vi "Dashboard Main.vi"() -> ()   [LabVIEW 2013]
uses:
  AnnieFramework/DoubleSolenoidAction.ctl
  AnnieFramework/CollectorAction.ctl
  AnnieFramework/CollectorWrapAction.ctl
  AnnieFramework/CatchAction.ctl
  AnnieFramework/AutoStates.ctl
  AnnieFramework/RollerAction.ctl
  AnnieFramework/AutoMode.ctl
  AnnieFramework/PassState.ctl
  AnnieFramework/HotGoalDetectType.ctl
  AnnieFramework/LowGoalState.ctl
  <vilib>/event_ctls.llb/eventvkey.ctl
  <vilib>/Rock Robotics/WPI/Dashboard/WPI_DashboardLogging Global.vi
  <vilib>/Utility/config.llb/Write Key (String).vi
  <vilib>/Utility/config.llb/Write Key (I32).vi
  KariFramework/CheckImageDistance.vi
  <vilib>/Utility/config.llb/NI_LVConfig.lvlib
panel:
  in  "Enable Vision":bool=TRUE
  out "Image Message":string="Timeout in Camera Communications"
  in  "Rec Mode":enum32{"Stop", "Record", "Playback"}(radio)
  in  "Dashboard Tab":T1(tab)
  out "Version":string
  in  "XBox":bool
  in  "DisableLCD":bool=TRUE
  out "GroundPassState":T2
  in  "DisableRollerOut":bool=TRUE
  out "FrontSonar":dbl
  out "ClosePressure":bool
  out "FarPressure":bool
  out "CatchState":T3
  out "CollectorWrapState":T4
  out "CollectorState":T5
  out "CollectorMotor":dbl
  out "ClapperState":T6
  out "RollerPneuState":T6
  out "FiringCylinder2":bool
  out "FiringCylinder1":bool
  out "Kicker":bool
  out "AutoDistanceDone?":bool
  out "BackSonar":dbl
  out "BottomLS":bool
  out "TopLS":bool
  in  "MaxMotorChange":dbl=1.5
  out "Error":bool
  out "Right Motor":dbl
  out "Left Motor":dbl
  in  "Camera Settings":T7={"Frame Rate"=30, "Compression"=30, "Size"=1} {"Frame Rate" scale=1.0..30.0; "Size" items=["640x480", "320x240", "160x120"]}
  out "Mode":T8(ring)=enum."Auto Disabled"
  out "Camera IP":string
  in  "DB Camera Config":bool
  out "fps":dbl format="%#.1g"
  out "Mbps":dbl format="%#.1g"
  out "Mbps 2":bool
  out "CloseDist":bool
  out "FarDist":bool
  out "Pressure":dbl
  out "RollerMotorState":T9
  in  "DisableServo":bool=TRUE
  out "ElevatedPassState":T2
  out "Arcade":bool
  out "TankDriveTime":dbl
  out "SonicShifter":bool
  out "StraightDrive":bool
  out "HalfDrive":bool
  out "ReverseDrive":bool
  out "Enum":T10
  in  "BallSettleWait":i32=130
  in  "PreCheckGoalWait":i32=260
  in  "Slowdown":dbl=36.0
  in  "Brake":dbl=12.0
  in  "DriveDistance":dbl=36.0
  in  "DriveMinTime":i32=2000
  in  "DriveTimeout":i32=5000
  out "WasHot?":bool
  out "DriveTimeOut":bool
  out "CheckGoalTimedOut?":bool
  out "ElapsedTime":u32
  out "StateTime":u32
  out "CurrentState":T11
  out "RaiseArmTimedOut":bool
  out "LowerArmTimedOut":bool
  out "IDMatched?":bool
  in  "AutoID":i32=3061
  in  "AutoMode":T12=enum."OneBallCollector"
  in  "WebcamStartTime (ms)":i32=2000
  out "WebcamMatched?":bool
  in  "SaveToDisk?":bool
  in  "WebcamImages":i32=1
  in  "ResetWebcam?":bool=TRUE
  out "WebcamImagesProcessed":i32
  in  "HotGoalType":T13
  out "ServoAngle":dbl
  in  "% Cutoff":dbl=0.5
  out "NumHot":i32
  out "NumProcessed":i32
  in  "NumSamples":i32=5
  out "ProcessImage?":bool
  in  "Finished?":bool
  in  "Hot?":bool
  in  "Score cutoff":dbl=0.5
  in  "Color System":u16(ring)=2 items=["RGB", "HSL", "HSV", "HSI"]
  out "Distance (ft)":dbl
  in  "Color Components":T14={"Hue"={112.0, 144.0}, "Sat"={202.0, 255.0}, "Val"={237.0, 255.0}} {"Val" scale=0.0..255.0; "Sat" scale=0.0..255.0; "Hue" scale=0.0..255.0 scale format="%#_3g"}
  out "LoopTime":u32
  in  "Calibrate?":bool
  in  "Reset?":bool
  in  "Test Slider":dbl(slide) scale=0.0..100.0 scale format="%#_3g"
  in  "On/Off":bool caption="Solenoid"
  in  "Test Name":u16(ring) items=["Select the test to run...", "Example Test", "-------------------------------", "List of tests is built in robot code.", "Replace with your own automated tests."]
  in  "Test Tree":string(tree)
  in  "Motor":cluster{"Value":dbl, "Enable":bool} {"Value" scale=-1.0..1.0 scale format="%#_3g"}
  out "Progress":T15 {"Test Progress" scale=0.0..100.0}
  in  "Rev/Fwd":cluster{"Forward":bool, "Reverse":bool}
  in  "Test Ring":u16(ring) items=["Auto", "Fixed indoor", "Fixed outdoor 1", "Fixed outdoor 2", "Fixed fluorescent 1", "Fixed fluorescent 2", "Hold current"]
  in  "Listbox":i32(listbox)
  out "Tree":string(tree)
  out "Timer":u32
  in  "CountdownStartTime":u32=10
  in  "AutoLength":u32=10
  in  "TeleopLength":u32=140
  out "Status":T16(ring)
  out "Errors":T17(array[cluster])
  in  "Reset":bool
  out "Camera Image":T18(plugin-control)
  # "DRIVE"
  # "GENERAL"
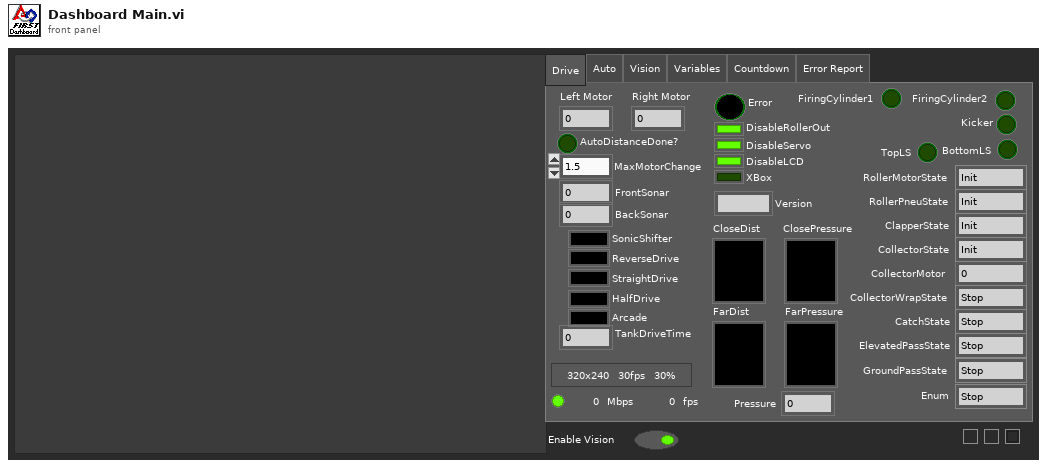
[diagram p1: front panel]
types:
  T1 = enum32{"Drive", "Auto", "Vision", "Test", "Checklist", "Variables", "Countdown", "Error Report"}
  T2 = typedef "PassState.ctl" = enum16{"Stop", "Pass"}
  T3 = typedef "CatchAction.ctl" = enum16{"Stop", "PreCatch", "Catch"}
  T4 = typedef "CollectorWrapAction.ctl" = enum16{"Stop", "PreCollect", "Collect"}
  T5 = typedef "CollectorAction.ctl" = enum16{"Init", "Raise", "Lower", "Stop", "GetStatus"}
  T6 = typedef "DoubleSolenoidAction.ctl" = enum16{"Init", "Middle", "In", "Out"}
  T7 = cluster{"Frame Rate":i32, "Compression":i32, "Size":u16}
  T8 = enum8{"Tele-Op Disabled", "Tele-Op Enabled", "Auto Disabled", "Auto Enabled", "Test Disabled", "Test Enabled", ""}
  T9 = typedef "RollerAction.ctl" = enum16{"Init", "Off", "Forward", "Reverse"}
  T10 = typedef "LowGoalState.ctl" = enum16{"Stop", "Shoot"}
  T11 = typedef "AutoStates.ctl" = enum16{"Init", "LowerArmCheckGoal", "DriveBack", "Collect", "StopCollect", "LiftArm", "RaiseServo", "Drive", "ShootCollectorUp", "RaiseArm", "ShootCollectorDown", "Rotate1", "Rotate2", "Stop"}
  T12 = typedef "AutoMode.ctl" = enum16{"OneBallFront", "OneBallCollector", "TwoBallNormal", "TwoBallHot"}
  T13 = typedef "HotGoalDetectType.ctl" = enum16{"VisionTarget", "Kinect"}
  T14 = cluster{"Hue":cluster{dbl, dbl}, "Sat":cluster{dbl, dbl}, "Val":cluster{dbl, dbl}}
  T15 = cluster{"Test Progress":u8, "Test Progress Text":string}
  T16 = enum8{"Disconnected", "E-Stop", "Disabled", "Enabled"}
  T17 = cluster{"status":bool, "code":i32, "location":string, "source":string}[]
  T18 = typedef "IMAQ Image.ctl" = refnum<image>
  T19 = enum32{"Drive", "Operation", "Auto", "Test", "Checklist", "Variables"}
  T20 = typedef "Image Type" = u32
  T21 = typedef "NI_LVConfig.lvlib/Config Data RefNum.ctl" = refnum<k1>
  T22 = cluster{"Digital Inputs":bool[], "Digital Outputs":bool[]}
  T23 = cluster{"Competition mode":bool, "Robot Link":bool, "Autonomous":bool, "Enabled":bool, "E-Stop":bool, "Simulated":bool, "TestMode":bool, "Docked Window":bool}
  T24 = typedef "CountdownAction.ctl" = enum16{"Start", "Reset", "Continue", "Idle"}
  T25 = cluster{"Boolean":bool, "Numeric":i32, "String":string, "String":string}[]
  T26 = cluster{cluster{dbl, dbl}, cluster{dbl, dbl}, cluster{dbl, dbl}}
  T27 = typedef "Sound Output Task ID.ctl" = u32
  T28 = typedef "eventvkey.ctl" = enum16{"ASCII", "Enter", "Return", "Shift", "Ctrl", "Alt", "Cmd", "Opt", "Caps", "NumLock", "Clear", "Break", "Up", "Down", "Left", "Right", "Insert", "Delete", "Home", "End", "PageUp", "PageDown", "Escape", "Help", "Pause", "ScrollLock", "F1", "F2", "F3", "F4", "F5", "F6", "F7", "F8", "F9", "F10", "F11", "F12", "F13", "F14", "F15", "F16", "F17", "F18", "F19", "F20", "F21", "F22", "F23", "F24", "Play", "VolumeUp", "VolumeDown", "Mute", "Two Byte Char"}
  T29 = cluster{"Image Size":bool, "Image Type":bool, "Pixel Value":bool, "ROI Information":bool, "Zoom Factor":bool}
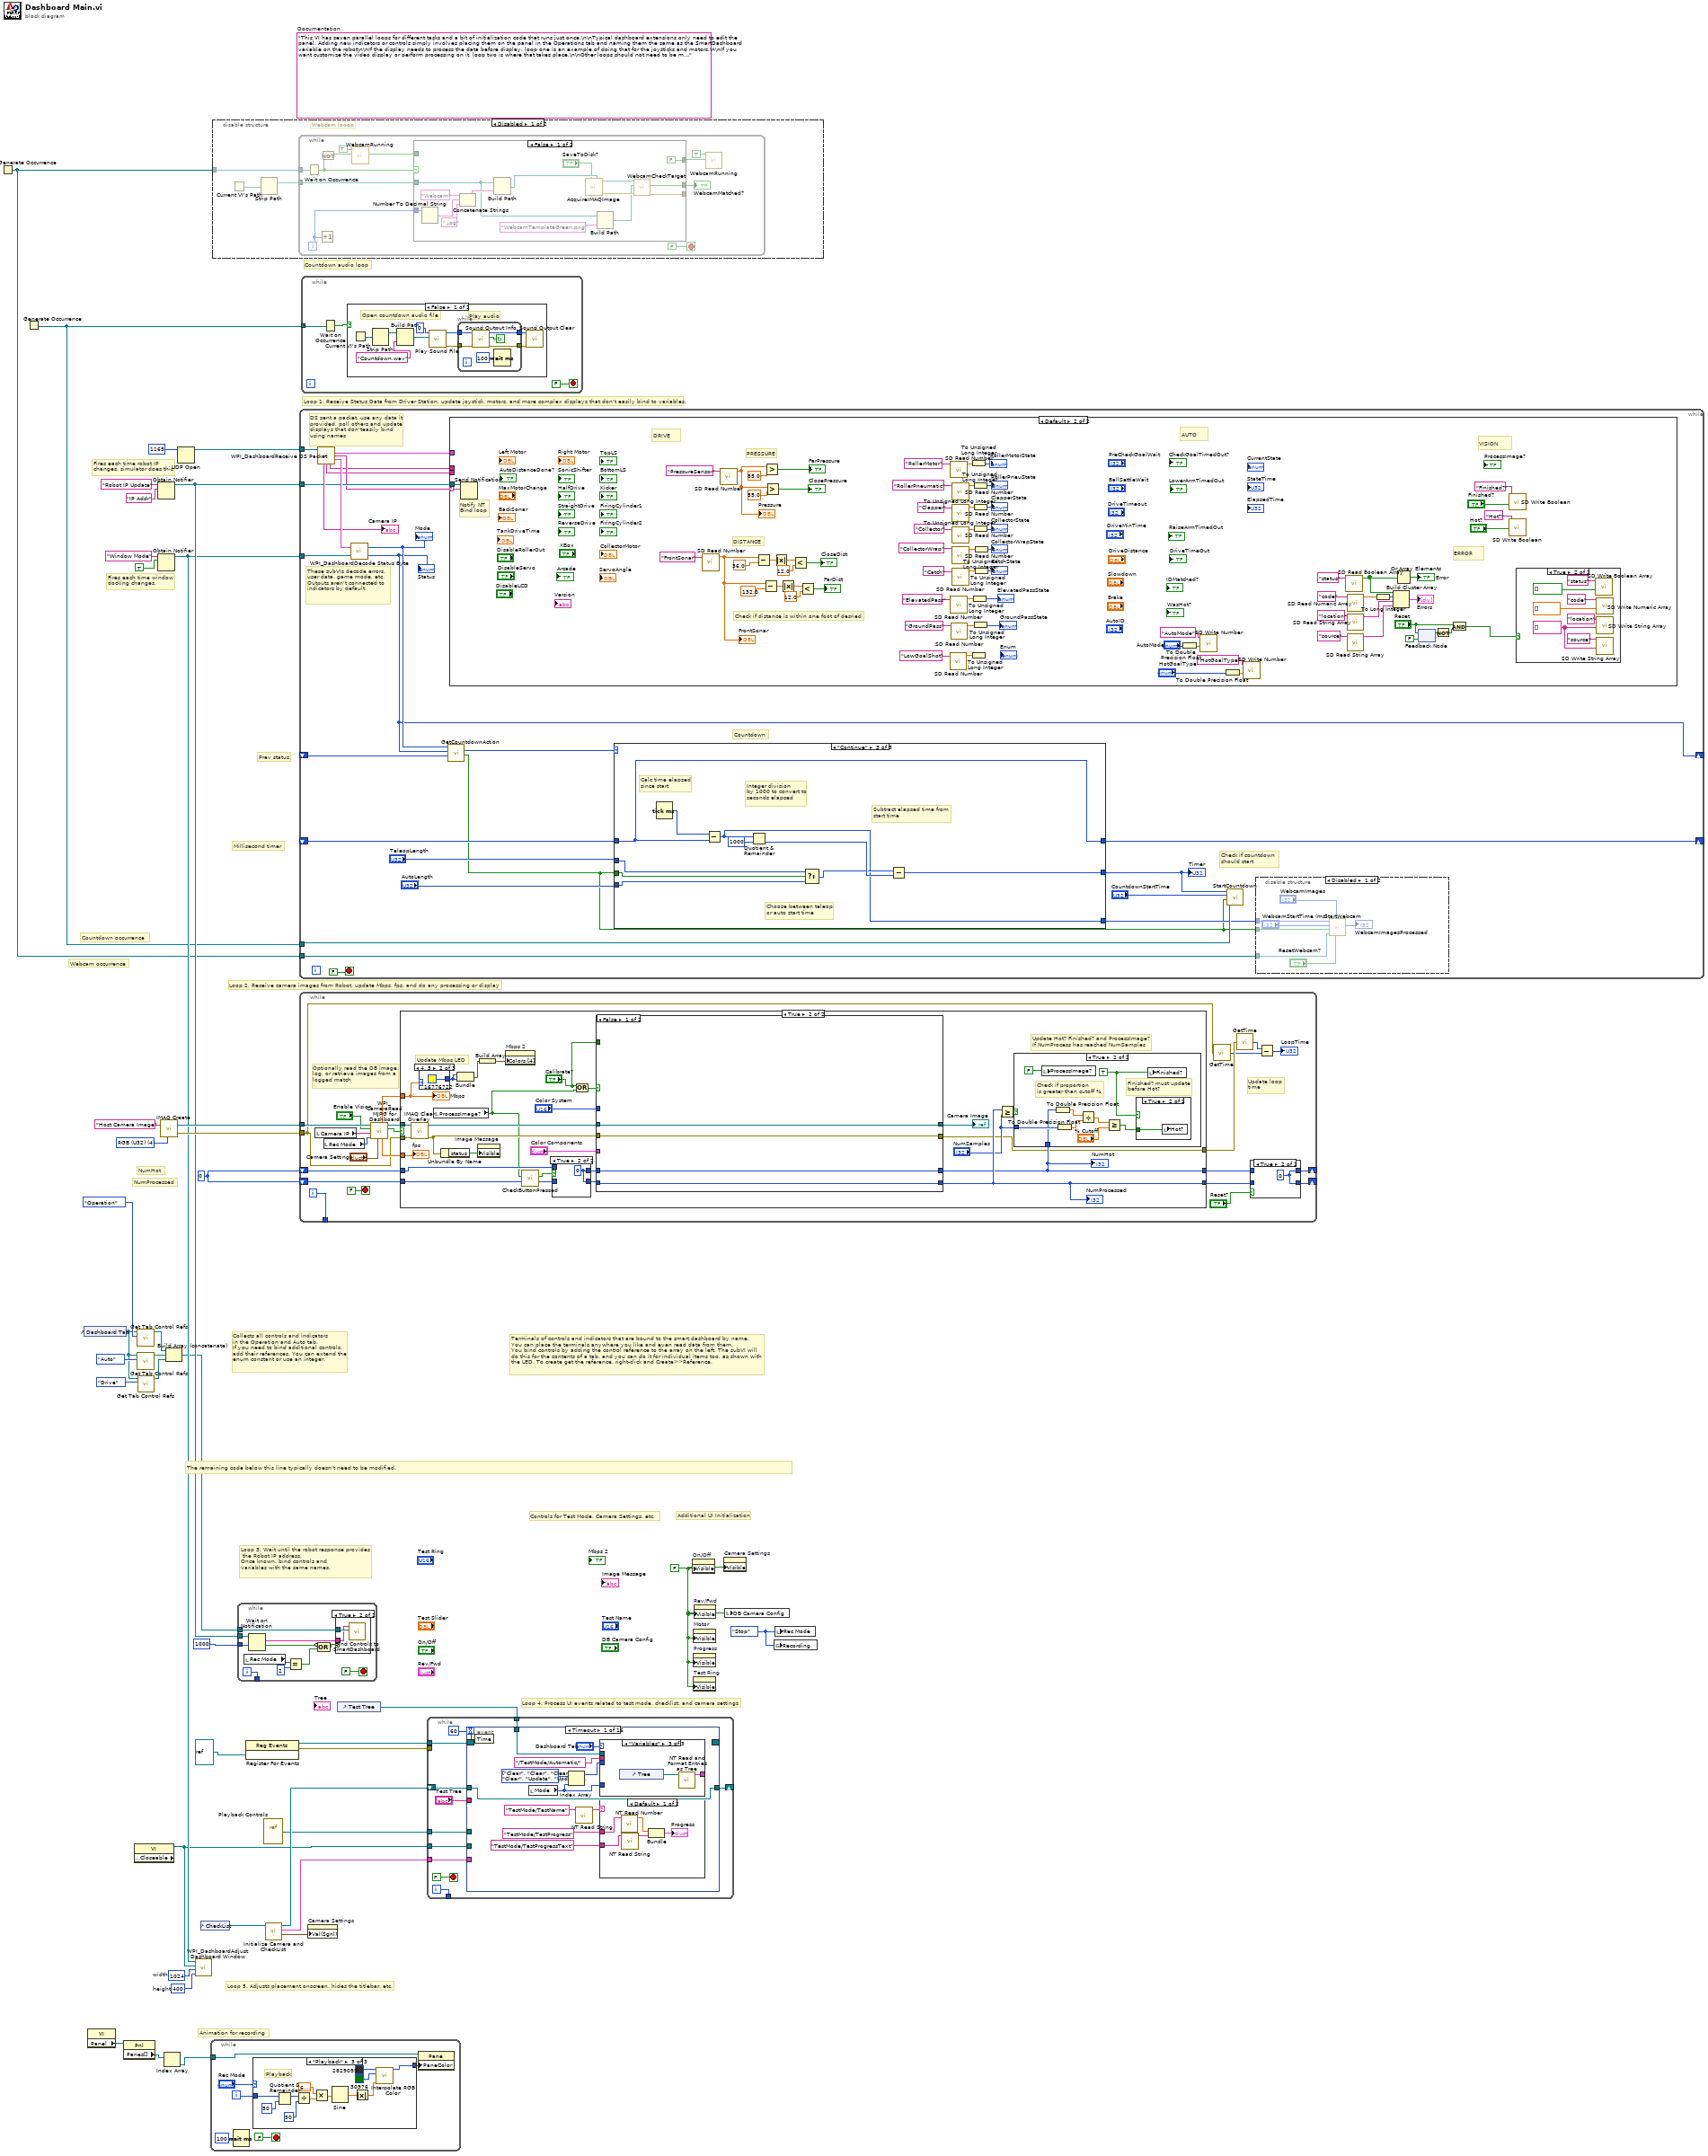
[diagram p0: block diagram]
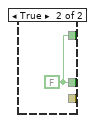
[diagram p2: hidden frame]
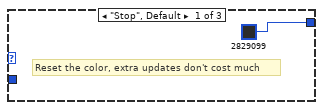
[diagram p5: hidden frame]
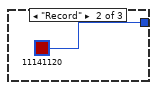
[diagram p6: hidden frame]
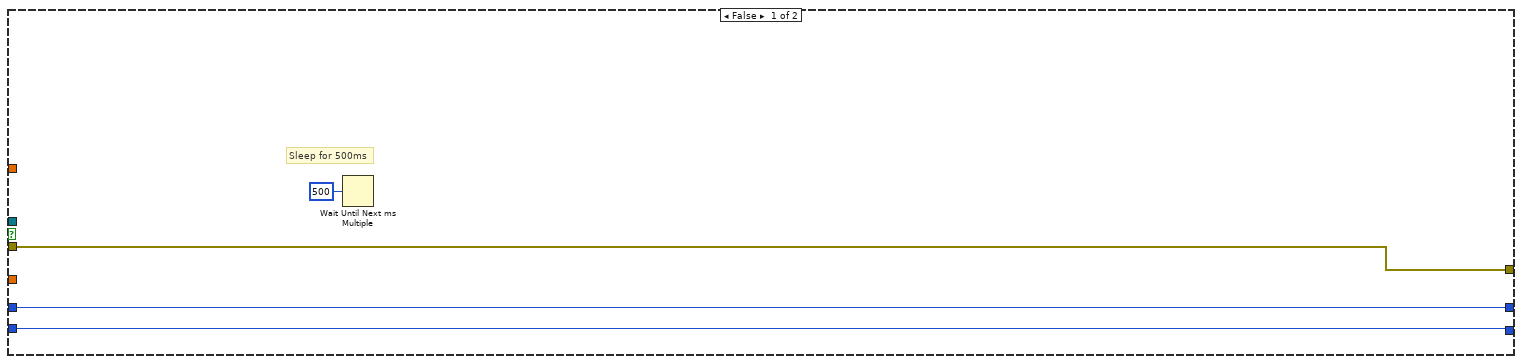
[diagram p9: hidden frame]
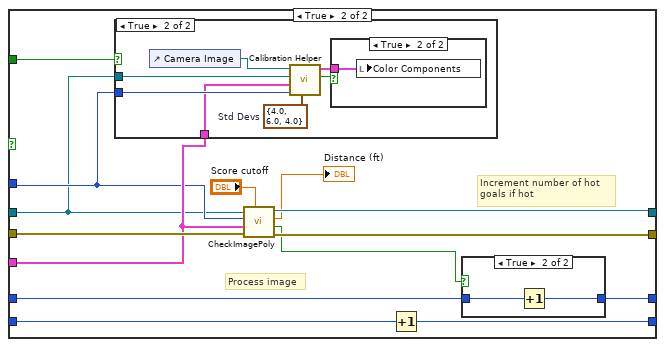
[diagram p13: hidden frame]
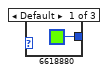
[diagram p17: hidden frame]
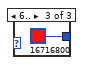
[diagram p18: hidden frame]
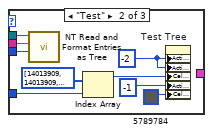
[diagram p20: hidden frame]
diagram:
  w3 = 0
  w12 = enum32{"Stop", "Record", "Playback"}."Stop" ("Rec Mode")
  w15 = 400  # height
  w16 = 1024  # width
  w29 = FALSE ("Visible")
  (unwired) "This VI has seven parallel loops for different tasks and a bit of initialization code that runs just once.\n\nTypical dashboard extensions only need to edit the panel. Adding new indicators or controls simply involves placing them on the panel in the Operations tab and naming them the same as the SmartDashboard variable on the robot\n\nIf the display needs to process the data before display, loop one is an example of doing that for the joysticks and motors.\n\nIf you want customize the video display or perform processing on it, loop two is where that takes place.\n\nOther loops should not need to be modified. They are pretty standard, and document the task they perform."  # Documentation
  w39 = T20 4 items=["Grayscale (U8)", "Grayscale (I16)", "Grayscale (SGL)", "Complex (CSG)", "RGB (U32)", "HSL (U32)", "RGB (U64)"] ("Image Type")
  # "Webcam occurrence"
  # "Countdown audio loop"
  # "Countdown occurrence"
  # "Millisecond timer"
  # "Prev status"
  # "NumProcessed"
  # "NumHot"
  # "Controls for Test Mode, Camera Settings, etc."
  # "Additional UI Initialization"
  # "Animation for recording"
  # "Fires each time robot IP\nchanges, simulator does this"
  # "Fires each time window\ndocking changes."
  # "Collects all controls and indicators\nin the Operation and Auto tab.\nIf you need to bind additional controls,\nadd their references. You can extend the\nenum constant or use an integer."
  # "The remaining code below this line typically doesn't need to be modified."
  # "Loop 4. Process UI events related to test mode, checklist, and camera settings"
  # "Terminals of controls and indicators that are bound to the smart dashboard by name.\nYou can place the terminals anywhere you like and even read data from them.\nYou bind controls by adding the control reference to the array on the left. The subVI will\ndo this for the contents of a tab, and you can do it for individual items too, as shown with\nthe LED. To create get the reference, right-click and Create>>Reference."
  # "Loop 3. Wait until the robot response provides\n the Robot IP address.\nOnce known, bind controls and\nvariables with the same names."
  # "Loop 5. Adjusts placement onscreen, hides the titlebar, etc."
  # "Loop 1. Receive Status Data from Driver Station, update joystick, motors, and more complex displays that don't easily bind to variables."
  # "Loop 2. Receive camera images from Robot, update Mbps, fps, and do any processing or display"
  n1 = Generate Occurrence() -> (w1:refnum<k4>)
  n2 = Generate Occurrence() -> (w2:refnum<k4>)
  n3 = control-ref of="Dashboard Tab"() -> (w5:refnum<vi>)
  n4 = property class="VI"() -> ("Panel"=w23:refnum<vi>)  [unwired: 2 in, 2 out]
  n5 = property class="Pnl"(reference=w23) -> ("Panes[]"=w24:refnum<vi>[])  [unwired: 1 in, 2 out]
  n6 = property class="VI" props=["Front Panel.Closeable"]() -> (reference out=w11:refnum<vi>)  [unwired: 2 in, 2 out]
  n7 = call <vilib>:"Get Tab Control Refs.vi"("Page Index"=T19."Operation" ("Dashboard Tab"), "TabControl in"=w5) -> ("ControlsOnPage"=w9:refnum<vi>[])  [unwired: 9 in]
  n8 = call <vilib>:"Get Tab Control Refs.vi"("Page Index"=T19."Auto" ("Dashboard Tab"), "TabControl in"=w5) -> ("ControlsOnPage"=w10:refnum<vi>[])  [unwired: 9 in]
  n9 = call <vilib>:"Get Tab Control Refs.vi"("Page Index"=T19."Drive" ("Dashboard Tab"), "TabControl in"=w5) -> ("ControlsOnPage"=w4:refnum<vi>[])  [unwired: 9 in]
  n10 = Obtain Notifier(name (unnamed)="Robot IP Update", notification data type="IP Addr" ("name (unnamed)")) -> (notifier out=w33:refnum<notifier>)  [unwired: 2 in, 2 out]
  n11 = Obtain Notifier(name (unnamed)="Window Mode", notification data type=TRUE) -> (notifier out=w14:refnum<notifier>)  [unwired: 2 in, 2 out]
  n12 = call "IMAQ Create"("Image Name"="Host Camera Image", "Image Type"=w39) -> ("New Image"=w37:T18, "error out"=w36:errorcluster)  [unwired: 2 in, 1 out]
  n13 = Index Array(array=w24) -> (element=w22:refnum<vi>)  [unwired: 1 in]
  n14 = Build Array (concatenate)(w9, w10, w4) -> (w8:refnum<vi>[])
  n15 = UDP Open(11:u16 1165 ("port")) -> (port=w40:refnum<k16>)  [unwired: 2 in, 4 out]
  n16 = call <vilib>:"WPI_DashboardAdjust Dashboard Window.vi"("height"=w15, "width"=w16, "reference in"=w11, "Notifier in"=w14) -> ()  [unwired: 8 in]
  n17 = control-ref of="CheckList"() -> (w13:refnum<vi>)
  n18 = while {
    tunnel: w22 -> [w43]
    i -> [w46]
    stop <- FALSE stop-if-true
    n19 = Wait (ms)(milliseconds to wait=u32 100) -> ()  [unwired: 1 out]
    n20 = case shown="\"Playback\"" "Rec Mode" {
      tunnel: w46 -> [_ _ w61]
      tunnel: [u32 2829099 ("Base Color") u32 11141120 ("Target Color") w50] -> w42
      frame "Stop", Default {
        # "Reset the color, extra updates don't cost much"
      }
      frame "Record" {
      }
      frame "Playback" {
        # "Playback"
        n21 = Quotient & Remainder(x=w61, y=u32 50 ("milliseconds to wait")) -> (x-y*floor(x/y)=w57:u32)  [unwired: 1 out]
        n22 = Divide(x=w57, y=u32 50 ("milliseconds to wait")) -> (x/y=w54:dbl)
        n23 = Multiply(x=6.283185307179586, y=w54) -> (x*y=w59:dbl)
        n24 = Sine(x=w59) -> (sin(x)=w58:dbl)
        n25 = Absolute Value(x=w58) -> (abs(x)=w51:dbl)
        n26 = call "Interpolate RGB Color.vi"("Proportion"=w51, "Target Color"=u32 30976, "Base Color"=u32 2829099) -> ("Result Color"=w50:u32)  [unwired: 8 in]
      }
    }
    n27 = property class="Pane"(reference=w43, "PaneColor"=w42) -> ()  [unwired: 1 in, 2 out]
  }
  n28 = disable-structure shown="Disabled" {
    disable-tunnel: w1 -> [w64 _]
    frame Disabled {
      # "Webcam looop"
      n29 = Current VI's Path() -> (path=w63:path)
      n30 = Strip Path(path=w63) -> (stripped path=w62:path)  [unwired: 1 out]
      n31 = while {
        tunnel: w64 -> [w75]
        tunnel: w62 -> [w72]
        i -> [w71]
        stop <- FALSE stop-if-true
        n32 = Wait on Occurrence(2:w75) -> (0:w69:bool)  [unwired: 2 in]
        n33 = Increment(x=w71) -> ()  [unwired: 1 out]
        n34 = Not(x=w69) -> (.not. x?=w68:bool)
        n35 = call "WebcamRunning"("NewValue"=w68, "Write?"=TRUE) -> ("CurrentValue"=w65:bool)  [unwired: 9 in]
        n36 = case shown="False" w69 {
          tunnel: [w88 _] -> _
          tunnel: [w87 w91] -> w73
          tunnel: w71 -> [w85 _]
          tunnel: w72 -> [w79 _]
          tunnel: [FALSE w91] -> w66
          tunnel: w65 -> [_ _]
          frame False {
            n37 = Number To Decimal String(number=w85) -> (decimal integer string=w84:string)  [unwired: 1 in]
            n38 = Concatenate Strings("Webcam", w84, ".jpg" ("string")) -> (w83:string)
            n39 = Build Path(base path=w79, name or relative path=w83) -> (appended path=w82:path)
            n40 = call "AcquireIMAQImage.vi"("ImagePath"=w82, "SaveToDisk?"="SaveToDisk?") -> ("error out"=w89:errorcluster, "ImageOut"=w90:T18)  [unwired: 8 in]
            n41 = Build Path(base path=w79, name or relative path="WebcamTemplateGreen.png") -> (appended path=w78:path)
            n42 = call "WebcamCheckTarget.vi"("error in"=w89, "TemplatePath"=w78, "ImageIn"=w90) -> ("error out"=w88:errorcluster, "MatchFound?"=w87:bool)  [unwired: 6 in, 1 out]
          }
          frame True {
            w91 = FALSE ("MatchFound?")
          }
        }
        "WebcamMatched?" <- w73
        n43 = call "WebcamRunning"("NewValue"=w66, "Write?"=TRUE) -> ()  [unwired: 9 in, 1 out]
      }
    }
    frame Enabled {
    }
  }
  n44 = while {
    tunnel: w8 -> [w102]
    tunnel: w33 -> [w100]
    tunnel: [w98] -> _
    tunnel: u32 1000 ("milliseconds to wait") -> [w97]
    i -> [w98]
    stop <- FALSE stop-if-true
    n45 = local read "Rec Mode"() -> (w93:enum32{"Stop", "Record", "Playback"})
    n46 = Wait on Notification(notifier=w100, timeout in ms (-1)=w97) -> (notification=w99:string, timed out?=w95:bool)  [unwired: 2 in, 2 out]
    n47 = Equal?(x=w93, y=u16 2 ("Rec Mode")) -> (x = y?=w94:bool)
    n48 = Compound Arithmetic op=OR(invert w95, w94) -> (w96:bool)
    n49 = case shown="True" w96 {
      tunnel: w102 -> [_ w104]
      tunnel: w99 -> [_ w103]
      frame False {
      }
      frame True {
        n50 = call <vilib>:"Bind Controls to SmartDashboard.vi"("Bound Control Refs"=w104, "Server IP Address"=w103) -> ()  [unwired: 10 in]
      }
    }
  }
  n51 = register-events(refnum<vi> refnum) -> (reference out=w20:refnum<event-registration>, error out=w19:errorcluster)  [unwired: 2 in]
  n52 = vi-ref "Playback Controls.vi"() -> (w21:refnum<vi>)
  n53 = call "Initialize Camera and CheckList.vi"("ListBox in"=w13) -> ("Cluster"=w27:cluster{"value":i32, "value":i32, "index":i32}, "Array"=w28:cluster{string[]}[], "File Refnum"=w26:T21)  [unwired: 8 in]
  n54 = while {
    tunnel: w40 -> [w126]
    tunnel: w33 -> [w123]
    tunnel: w14 -> [w125]
    shift-right: [w117] -> _
    shift-left: _ -> [w116]
    shift-right: [w114] -> _
    shift-left: _ -> [w113]
    tunnel: w2 -> [w108]
    tunnel: w1 -> [w105]
    stop <- FALSE stop-if-true
    # "Check if countdown\nshould start"
    # "Countdown"
    # "DS sent a packet. use any data it\nprovided, poll others and update\ndisplays that don'teasily bind\nusing names"
    # "These subVIs decode errors, user data, game mode, etc.\nOutputs aren't connected to indicators by default"
    n55 = call <vilib>:"WPI_DashboardReceive DS Packet.vi"("Recv Socket"=w126) -> ("Driver Station"=w119:T22, "Robot IP Address"=w122:string, "Status"=w127:T23, "Camera IP Address"=→"Camera IP":string, "Low Priority User Data"=w121:string, "High Priority User Data"=w120:string)  [unwired: 1 in, 8 out]
    n56 = call <vilib>:"WPI_DashboardDecode Status Byte.vi"("Window Mode Notifier"=w125, "Status"=w127) -> ("Status"=w117:T16, "Mode"=w118:T8)
    "Mode" <- w118
    "Status" <- w117
    n57 = call "GetCountdownAction.vi"("PrevStatus"=w116, "CurrentStatus"=w117, "CurrentMode"=w118) -> ("Teleop?"=w106:bool, "Action"=w115:T24)  [unwired: 7 in]
    n58 = case shown="Default" w122 {
      selector: w122 -> [_ w224]
      tunnel: w123 -> [_ w225]
      tunnel: w121 -> [_ _]
      tunnel: w120 -> [_ _]
      tunnel: w119 -> [_ _]
      frame "0.0.0.0" {
        # "DS not sending packets, or no robot exists yet.\nDon't poll the variables"
      }
      frame Default {
        # "Check if distance is within one foot of desried"
        # "ERROR"
        # "DISTANCE"
        # "PRESSURE"
        # "VISION"
        # "AUTO"
        # "DRIVE"
        # "Notify NT\nBind loop"
        n59 = Send Notification(notification=w224, notifier=w225) -> ()  [unwired: 1 in, 2 out]
        n60 = call <vilib>:"SD Read Number.vi"("Name"="FrontSonar") -> ("Numeric"=w172:dbl)  [unwired: 8 in, 2 out]
        "FrontSonar" <- w172
        n61 = call <vilib>:"SD Read Number.vi"("Name"="PressureSensor") -> ("Numeric"=w171:dbl)  [unwired: 8 in, 2 out]
        "Pressure" <- w171
        n62 = Subtract(x=w172, y=36.0) -> (x-y=w181:dbl)
        n63 = Subtract(x=w172, y=132.0) -> (x-y=w175:dbl)
        n64 = Greater?(x=w171, y=85.0) -> (0:→"FarPressure":bool)
        n65 = Greater?(x=w171, y=55.0) -> (0:→"ClosePressure":bool)
        n66 = Absolute Value(x=w181) -> (abs(x)=w180:dbl)
        n67 = Absolute Value(x=w175) -> (abs(x)=w176:dbl)
        n68 = Less?(x=w180, y=12.0) -> (x < y?=→"CloseDist":bool)
        n69 = Less?(x=w176, y=12.0) -> (x < y?=→"FarDist":bool)
        n70 = call <vilib>:"SD Read Number.vi"("Name"="LowGoalShot") -> ("Numeric"=w154:dbl)  [unwired: 8 in, 2 out]
        n71 = call <vilib>:"SD Read Number.vi"("Name"="RollerMotor") -> ("Numeric"=w169:dbl)  [unwired: 8 in, 2 out]
        n72 = call <vilib>:"SD Read Number.vi"("Name"="ElevatedPass") -> ("Numeric"=w163:dbl)  [unwired: 8 in, 2 out]
        n73 = call <vilib>:"SD Read Number.vi"("Name"="GroundPass") -> ("Numeric"=w162:dbl)  [unwired: 8 in, 2 out]
        n74 = call <vilib>:"SD Read Number.vi"("Name"="RollerPneumatic") -> ("Numeric"=w202:dbl)  [unwired: 8 in, 2 out]
        n75 = call <vilib>:"SD Read Number.vi"("Name"="Clapper") -> ("Numeric"=w200:dbl)  [unwired: 8 in, 2 out]
        n76 = call <vilib>:"SD Read Number.vi"("Name"="Collector") -> ("Numeric"=w197:dbl)  [unwired: 8 in, 2 out]
        n77 = call <vilib>:"SD Read Number.vi"("Name"="CollectorWrap") -> ("Numeric"=w194:dbl)  [unwired: 8 in, 2 out]
        n78 = call <vilib>:"SD Read Number.vi"("Name"="Catch") -> ("Numeric"=w191:dbl)  [unwired: 8 in, 2 out]
        n79 = To Unsigned Long Integer(number=w169) -> (unsigned 32bit integer=→"RollerMotorState":u32)
        n80 = To Unsigned Long Integer(number=w154) -> ()  [unwired: 1 out]
        n81 = To Unsigned Long Integer(number=w163) -> (unsigned 32bit integer=→"ElevatedPassState":u32)
        n82 = To Unsigned Long Integer(number=w202) -> (unsigned 32bit integer=→"RollerPneuState":u32)
        n83 = To Unsigned Long Integer(number=w200) -> (unsigned 32bit integer=→"ClapperState":u32)
        n84 = To Unsigned Long Integer(number=w162) -> (unsigned 32bit integer=→"GroundPassState":u32)
        n85 = To Unsigned Long Integer(number=w197) -> (unsigned 32bit integer=→"CollectorState":u32)
        n86 = To Unsigned Long Integer(number=w194) -> (unsigned 32bit integer=→"CollectorWrapState":u32)
        n87 = To Unsigned Long Integer(number=w191) -> (unsigned 32bit integer=→"CatchState":u32)
        n88 = To Double Precision Float(number="AutoMode") -> (double precision float=w165:dbl)
        n89 = call <vilib>:"SD Write Number.vi"("Numeric"=w165, "Name"="AutoMode") -> ()  [unwired: 8 in, 2 out]
        n90 = To Double Precision Float(number="HotGoalType") -> (double precision float=w158:dbl)
        n91 = call <vilib>:"SD Write Number.vi"("Numeric"=w158, "Name"="HotGoalType") -> ()  [unwired: 8 in, 2 out]
        n92 = call <vilib>:"SD Read Boolean Array.vi"("Name"="status") -> ("Boolean Array"=w213:bool[])  [unwired: 8 in, 2 out]
        n93 = call <vilib>:"SD Read Numeric Array.vi"("Name"="code") -> ("Numeric Array"=w212:dbl[])  [unwired: 8 in, 2 out]
        n94 = call <vilib>:"SD Read String Array.vi"("Name"="location") -> ("String Array"=w211:string[])  [unwired: 9 in, 1 out]
        n95 = call <vilib>:"SD Read String Array.vi"("Name"="source") -> ("String Array"=w210:string[])  [unwired: 9 in, 1 out]
        n96 = To Long Integer(number=w212) -> (32bit integer=w218:i32[])
        n97 = Build Cluster Array(w213, w218, w211, w210) -> (→"Errors":T25)
        n98 = Or Array Elements(Boolean array=w213) -> (logical OR=→"Error":bool)
        n99 = feedback #1(FALSE ("Reset")) -> (w221:bool)
        n100 = feedback-in #1("Reset") -> ()
        n101 = Not(x=w221) -> (.not. x?=w220:bool)
        n102 = And(x="Reset", y=w220) -> (x .and. y?=w219:bool)
        n103 = call <vilib>:"SD Write Boolean.vi"("Boolean"="Finished?", "Name"="Finished?") -> ()  [unwired: 8 in, 2 out]
        n104 = call <vilib>:"SD Write Boolean.vi"("Boolean"="Hot?", "Name"="Hot?") -> ()  [unwired: 8 in, 2 out]
        n105 = case shown="True" w219 {
          frame False {
          }
          frame True {
            w226 = string[] [] ("String Array")
            n106 = call <vilib>:"SD Write Boolean Array.vi"("Boolean Array"=bool[] [], "Name"="status") -> ()  [unwired: 8 in, 2 out]
            n107 = call <vilib>:"SD Write Numeric Array.vi"("Numeric Array"=dbl[] [], "Name"="code") -> ()  [unwired: 8 in, 2 out]
            n108 = call <vilib>:"SD Write String Array.vi"("String Array"=w226, "Name"="location") -> ()  [unwired: 8 in, 2 out]
            n109 = call <vilib>:"SD Write String Array.vi"("String Array"=w226, "Name"="source") -> ()  [unwired: 8 in, 2 out]
          }
        }
      }
    }
    n110 = case shown="\"Continue\"" w115 {
      tunnel: "TeleopLength" -> [w138 _ w151]
      tunnel: "AutoLength" -> [w137 _ w150]
      tunnel: [w141 w142 w149] -> w110
      tunnel: [w140 w143 w148] -> w114
      tunnel: w113 -> [_ w143 w148]
      tunnel: w106 -> [w139 _ w152]
      tunnel: [u32 0 ("millisecond timer value") w142 w144] -> w107
      frame "Start", Default {
        # "Choose between auto and teleop start times"
        n111 = Select(t=w138, s=w139, f=w137) -> (s? t:f=w141:u32)
        n112 = Tick Count (ms)() -> (millisecond timer value=w140:u32)
      }
      frame "Reset", "Idle" {
        w142 = u32 0 ("AutoStartTime")
      }
      frame "Continue" {
        # "Subtract elapsed time from\nstart time"
        # "Choose between teleop\nor auto start time"
        # "Integer division\nby 1000 to convert to\nseconds elapsed"
        # "Calc time elapsed\nsince start"
        n113 = Tick Count (ms)() -> (millisecond timer value=w145:u32)
        n114 = Subtract(x=w145, y=w148) -> (x-y=w144:u32)
        n115 = Quotient & Remainder(x=w144, y=u32 1000) -> (floor(x/y)=w147:u32)  [unwired: 1 out]
        n116 = Select(t=w151, s=w152, f=w150) -> (s? t:f=w146:u32)
        n117 = Subtract(x=w146, y=w147) -> (x-y=w149:u32)
      }
    }
    "Timer" <- w110
    n118 = call "StartCountdown.vi"("CountdownOccurrence"=w108, "Teleop?"=w106, "CountdownStartTime"="CountdownStartTime", "Time"=w110) -> ()  [unwired: 8 in]
    n119 = disable-structure shown="Disabled" {
      disable-tunnel: w107 -> [w135 _]
      disable-tunnel: w106 -> [w133 _]
      disable-tunnel: w105 -> [w132 _]
      frame Disabled {
        n120 = call "StartWebcam.vi"("ResetWebcam?"="ResetWebcam?", "NumWebcamImages"="WebcamImages", "WebcamOccurrence"=w132, "Teleop?"=w133, "WebcamStartTime (ms)"="WebcamStartTime (ms)", "ElapsedTime (ms)"=w135) -> ("WebcamImagesProcessed"=→"WebcamImagesProcessed":i32)  [unwired: 5 in]
      }
      frame Enabled {
      }
    }
  }
  n121 = while {
    tunnel: w37 -> [w253]
    tunnel: w36 -> [w238]
    tunnel: [w254] -> _
    shift-right: [w233] -> _
    shift-left: w3 -> [w243]
    shift-right: [w234] -> _
    shift-left: w3 -> [w244]
    i -> [w254]
    stop <- FALSE stop-if-true
    # "Update loop\ntime"
    # "Optionally read the DB image,\nlog, or retrieve images from a\nlogged match"
    n122 = local read "Camera IP"() -> (w246:string)
    n123 = local read "Rec Mode"() -> (w245:enum32{"Stop", "Record", "Playback"})
    n124 = call <vilib>:"WPI_CameraRead MJPG for Dashboard.vi"("Camera Settings"="Camera Settings", "Rec Mode"=w245, "Camera IP"=w246, "Enable"="Enable Vision", "Refnum in"=w253) -> ("Active"=w250:bool, "Refnum out"=w252:T18, "FPS"=w249:dbl, "Bandwidth (Mbps)"=w248:dbl)  [unwired: 3 in]
    n125 = case shown="True" w250 {
      tunnel: w252 -> [_ w284]
      tunnel: w248 -> [_ w283]
      tunnel: w249 -> [_ w282]
      tunnel: w244 -> [w260 w272]
      tunnel: w243 -> [w261 w271]
      tunnel: [w261 w277] -> w236
      tunnel: [w260 w276] -> w235
      tunnel: [w259 w274] -> w241
      tunnel: w238 -> [w259 w273]
      frame False {
        # "Sleep for 500ms"
        n126 = Wait Until Next ms Multiple(millisecond multiple=u32 500) -> ()  [unwired: 1 out]
      }
      frame True {
        # "Update Hot? Finished? and ProcessImage?\nIf NumProcess has reached NumSamples"
        # "Update Mbps LED"
        n127 = call "IMAQ Clear Overlay"("error in (no error)"=w273, "Image"=w284) -> ("error out"=w279:errorcluster, "Image Out"=w281:T18)  [unwired: 1 in, 7 out]
        n128 = case shown="4, 5" w283 {
          tunnel: [u32 6618880 ("Color Box") u32 16776722 ("Color Box") u32 16716800 ("Color Box")] -> w285
          frame Default {
          }
          frame 4, 5 {
          }
          frame 6.. {
          }
        }
        n129 = local read "ProcessImage?"() -> (w264:bool)
        n130 = Unbundle By Name(w279) -> ("status"=w288:bool)
        n131 = Bundle("Color Box"=w285, "Color Box"=w285) -> (w287:cluster{"Color Box":u32, "Color Box":u32})  [unwired: 1 out]
        n132 = property on="Image Message" class="Str"("Visible"=w288) -> ()  [unwired: 2 in, 2 out]
        n133 = Build Array(w287) -> (w286:cluster{"Color Box":u32, "Color Box":u32}[])
        n134 = property on="Mbps 2" class="Bool (strict)"("Colors [4]"=w286) -> ()  [unwired: 2 in, 2 out]
        n135 = call "CheckButtonPressed.vi"("Button"=w264) -> ("Pressed?"=w268:bool)  [unwired: 9 in, 1 out]
        n136 = case shown="True" w268 {
          tunnel: w272 -> [w290 _]
          tunnel: w271 -> [w289 _]
          tunnel: [w290 w291] -> w270
          tunnel: [w289 w291] -> w269
          frame False {
          }
          frame True {
            w291 = 0
          }
        }
        n137 = Or(x="Calibrate?", y=w264) -> (x .or. y?=w265:bool)
        n138 = case shown="False" w265 {
          tunnel: w281 -> [w302 w307]
          tunnel: [w302 w316] -> w280
          tunnel: w270 -> [w304 w313]
          tunnel: w269 -> [w305 w315]
          tunnel: w279 -> [w303 w318]
          tunnel: [w303 w317] -> w274
          tunnel: [w305 w314] -> w277
          tunnel: [w304 w312] -> w276
          tunnel: "Color Components" -> [_ w309]
          tunnel: "Color System" -> [_ w308]
          tunnel: "Calibrate?" -> [_ w306]
          frame False {
          }
          frame True {
            # "Process image"
            # "Increment number of hot\ngoals if hot"
            n139 = case shown="True" w306 {
              tunnel: w308 -> [_ w325]
              tunnel: w309 -> [_ w324]
              tunnel: w307 -> [_ w323]
              frame False {
              }
              frame True {
                w326 = cluster{"Hue":dbl, "Sat":dbl, "Val":dbl} {"Hue"=4.0, "Sat"=6.0, "Val"=4.0}  # Std Devs
                n140 = control-ref of="Camera Image"() -> (w322:refnum<vi>)
                n141 = call "Calibration Helper.vi"("Std Devs"=w326, "Color Mode"=w325, "Color Components"=w324, "Image"=w323, "Image Ctl Refnum"=w322) -> ("Changed"=w320:bool, "output color"=w321:T26)  [unwired: 5 in]
                n142 = case shown="True" w320 {
                  tunnel: w321 -> [_ w327]
                  frame False {
                  }
                  frame True {
                    n143 = local write "Color Components"(w327) -> ()
                  }
                }
              }
            }
            n144 = call-poly "CheckImagePoly.vi"("Score cutoff"="Score cutoff", "error in"=w318, "Color Components"=w309, "Color System"=w308, "Image"=w307) -> ("error out"=w317:errorcluster, "Hot?"=w310:bool, "Distance (ft)"=→"Distance (ft)":dbl, "Image out"=w316:T18)  [unwired: 3 in]
            n145 = Increment(x=w315) -> (x+1=w314:i32)
            n146 = case shown="True" w310 {
              tunnel: w313 -> [w328 w330]
              tunnel: [w328 w329] -> w312
              frame False {
              }
              frame True {
                n147 = Increment(x=w330) -> (x+1=w329:i32)
              }
            }
          }
        }
        "Camera Image" <- w280
        "NumHot" <- w276
        "NumProcessed" <- w277
        n148 = Greater Or Equal?(x=w277, y="NumSamples") -> (x >= y?=w278:bool)
        n149 = case shown="True" w278 {
          tunnel: w276 -> [_ w299]
          tunnel: "NumSamples" -> [_ w300]
          frame False {
          }
          frame True {
            w292 = TRUE ("Finished?")
            # "Finished? must update\nbefore Hot?"
            # "Check if proportion\nis greater than cutoff %"
            n150 = local write "ProcessImage?"(FALSE ("ProcessImage?")) -> ()
            n151 = To Double Precision Float(number=w299) -> (double precision float=w297:dbl)
            n152 = To Double Precision Float(number=w300) -> (double precision float=w298:dbl)
            n153 = Divide(x=w297, y=w298) -> (x/y=w296:dbl)
            n154 = Greater Or Equal?(x=w296, y="% Cutoff") -> (x >= y?=w294:bool)
            n155 = case shown="True" w292 {
              tunnel: w294 -> [_ w301]
              frame False {
              }
              frame True {
                n156 = local write "Hot?"(w301) -> ()
              }
            }
            n157 = local write "Finished?"(w292) -> ()
          }
        }
        "Mbps" <- w283
        "fps" <- w282
      }
    }
    n158 = call "GetTime.vi"("error in"=w238) -> ("Time"=w240:u32)
    n159 = call "GetTime.vi"("error in"=w241) -> ("Time"=w242:u32)
    n160 = case shown="True" "Reset?" {
      tunnel: w236 -> [w256 _]
      tunnel: w235 -> [w257 _]
      tunnel: [w257 w258] -> w234
      tunnel: [w256 w258] -> w233
      frame False {
      }
      frame True {
        w258 = 0
      }
    }
    n161 = Subtract(x=w242, y=w240) -> (x-y=→"LoopTime":u32)
  }
  n162 = while {
    tunnel: w2 -> [w334]
    stop <- FALSE stop-if-true
    n163 = Wait on Occurrence(2:w334) -> (0:w336:bool)  [unwired: 2 in]
    n164 = case shown="False" w336 {
      frame False {
        # "Play audio"
        # "Open countdown audio file"
        n165 = Current VI's Path() -> (path=w345:path)
        n166 = Strip Path(path=w345) -> (stripped path=w344:path)  [unwired: 1 out]
        n167 = Build Path(base path=w344, name or relative path="Countdown.wav") -> (appended path=w342:path)
        n168 = call <vilib>:"Play Sound File.vi"("path"=w342, "device ID"=u32 0) -> ("error out"=w340:errorcluster, "task ID"=w339:T27)  [unwired: 8 in]
        n169 = while {
          tunnel: w340 -> [w346]
          tunnel: w339 -> [w350]
          tunnel: [w349] -> w338
          tunnel: [w347] -> w337
          stop <- w348 continue-if-true
          n170 = call <vilib>:"Sound Output Info.vi"("error in (no error)"=w346, "task ID"=w350) -> ("error out"=w347:errorcluster, "is playing?"=w348:bool, "task ID out"=w349:T27)  [unwired: 6 in, 1 out]
          n171 = Wait (ms)(milliseconds to wait=u32 100) -> ()  [unwired: 1 out]
        }
        n172 = call <vilib>:"Sound Output Clear.vi"("error in (no error)"=w337, "task ID"=w338) -> ()  [unwired: 9 in, 1 out]
      }
      frame True {
      }
    }
  }
  n173 = property on="Camera Settings" class="Clust (strict)"("Val(Sgnl)"=w27) -> ()  [unwired: 2 in, 2 out]
  n174 = control-ref of="Test Tree"() -> (w25:refnum<vi>)
  n175 = while {
    tunnel: w28 -> [w359]
    shift-right: [w358] -> _
    shift-left: w26 -> [w357]
    tunnel: [w356] -> _
    tunnel: w25 -> [w355]
    tunnel: w21 -> [w354]
    tunnel: w20 -> [w353]
    tunnel: w19 -> [_]
    tunnel: w11 -> [w352]
    i -> [w356]
    stop <- FALSE stop-if-true
    n176 = event shown="[0] Timeout" {
      selector: w353 -> [_ _ _ _ _ _ _ _ _ _ _ _ _ _ _ _]
      dyn-events: [_ _ _ _ _ _ _ _ _ _ _ _ _ w597 _ _] -> _
      timeout: u32 60 ("milliseconds to wait") -> [_ _ _ _ _ _ _ _ _ _ _ _ _ _ _ _]
      tunnel: w355 -> [w369 _ _ _ _ _ _ _ _ _ _ _ _ _ _ _]
      tunnel: "Test Tree" -> [_ _ _ _ _ _ _ _ w566 w574 w576 w580 w588 _ _ _]
      tunnel: w359 -> [_ w393 _ _ _ _ w530 w560 _ _ _ _ _ _ _ _]
      tunnel: [w363 w392 w491 w496 w504 w516 w529 w553 w565 w572 w575 w579 w587 w599 w613 w614] -> w358
      tunnel: w357 -> [w363 w392 w491 w496 w504 w516 w528 w553 w565 w572 w575 w579 w587 w599 w613 w614]
      tunnel: w354 -> [_ _ _ _ _ _ _ _ _ _ _ _ _ w600 _ w617]
      tunnel: w352 -> [_ _ _ _ _ _ _ _ _ _ _ _ _ w595 _ _]
      event Timeout {
        w368 = enum16{"Update", "Clear"}[] [enum."Clear", enum."Clear", enum."Clear", enum."Clear", enum."Update", enum."Update", enum."Clear"] items=["Update", "Clear"]
        n177 = event-data() -> ()  [unwired: 1 in, 1 out]
        n178 = local read "Mode"() -> (w366:T8)
        n179 = Index Array(array=w368, index=w366) -> (element=w367:enum16{"Update", "Clear"})
        n180 = call <vilib>:"NT Read String.vi"("Name"="TestMode/TestName") -> ("String"=w372:string)  [unwired: 9 in, 1 out]
        n181 = case shown="\"Variables\"" "Dashboard Tab" {
          tunnel: w369 -> [_ w382 _]
          tunnel: "/TestMode/Automatic/" ("Name Pattern") -> [_ w381 _]
          tunnel: w367 -> [_ w380 _]
          tunnel: w366 -> [_ w378 _]
          tunnel: [_ _ w384] -> _
          frame "Auto", Default {
          }
          frame "Test" {
            w377 = -2 ("Active Item:Row Number")
            n182 = call <vilib>:"NT Read and Format Entries as Tree.vi"("Operation"=w380, "Name Pattern"=w381, "Tree Refnum"=w382) -> ()  [unwired: 7 in, 2 out]
            n183 = Index Array(array=u32[] [14013909, 14013909, 14013909, 14013909, 14013909, 16777215, 14013909], index=w378) -> (element=w376:u32)
            n184 = property on="Test Tree" class="Tree (strict)"("Active Item Row Number"=w377, "ActiveColNum"=w377, "CellBG"=w376, "Active Item Row Number"=-1 ("Active Item:Row Number"), "CellBG"=u32 5789784 ("Color Box")) -> ()  [unwired: 2 in, 2 out]
          }
          frame "Variables" {
            n185 = control-ref of="Tree"() -> (w383:refnum<vi>)
            n186 = call <vilib>:"NT Read and Format Entries as Tree.vi"("Tree Refnum"=w383) -> ("Formatted Strings"=w384:cluster{"Name":string, "Value":string}[])  [unwired: 9 in, 1 out]
          }
        }
        n187 = case shown="Default" w372 {
          tunnel: "TestMode/TestProgress" ("Name") -> [w386 _]
          tunnel: "TestMode/TestProgressText" ("Name") -> [w385 _]
          frame Default {
            n188 = call <vilib>:"NT Read Number.vi"("Name"=w386) -> ("Numeric"=w387:dbl)  [unwired: 9 in, 1 out]
            n189 = call <vilib>:"NT Read String.vi"("Name"=w385) -> ("String"=w388:string)  [unwired: 9 in, 1 out]
            n190 = Bundle("Numeric"=w387, "String"=w388) -> (→"Progress":cluster{"Numeric":dbl, "String":string})  [unwired: 1 in]
          }
          frame "" {
            n191 = property on="Progress" class="Clust (strict)"("Visible"=FALSE) -> ()  [unwired: 2 in, 2 out]
            n192 = local write "Test Name"(u16 0) -> ()
          }
        }
      }
      event "Test Tree": Value Change {
        # "Show appropriate\ncontrols"
        n193 = event-data() -> ("CtlRef"=w396:refnum<vi>, "NewVal"=w394:string)  [unwired: 1 in]
        n194 = call <vilib>:"WPI_UtilitiesGetTreeIOName.vi"("NewVal"=w394, "TreeControl in"=w396) -> ("I/O Name"=w397:string)  [unwired: 9 in]
        n195 = case shown="\"Camera\"" w397 {
          selector: w397 -> [_ w404 _ w422 w431 _]
          tunnel: w394 -> [_ _ w419 w421 _ w438]
          tunnel: w393 -> [_ _ _ _ _ w437]
          frame Default {
            w399 = FALSE ("Visible")
            w398 = FALSE ("Visible")
            n196 = property on="Motor" class="Clust (strict)"("Visible"=w398) -> ()  [unwired: 2 in, 2 out]
            n197 = property on="Test Ring" class="Ring (strict)"("Visible"=w398) -> ()  [unwired: 2 in, 2 out]
            n198 = property on="Rev/Fwd" class="Clust (strict)"("Visible"=w399) -> ()  [unwired: 2 in, 2 out]
            n199 = property on="On/Off" class="Bool (strict)"("Visible"=w399) -> ()  [unwired: 2 in, 2 out]
            n200 = property on="Test Slider" class="Slide (strict)"("Visible"=w399) -> ()  [unwired: 2 in, 2 out]
          }
          frame "Motor", "PWM" {
            w405 = FALSE ("Visible")
            n201 = case shown="\"Motor\", Default" w404 {
              tunnel: [1.0 ("Value") -1.0 ("Value")] -> w403
              tunnel: [255.0 ("Value") 1.0 ("Value")] -> w402
              tunnel: [128.0 ("Value") 0.0 ("Value")] -> w401
              tunnel: [64.0 ("Value") 0.5 ("Value")] -> w400
              frame "PWM" {
              }
              frame "Motor", Default {
              }
            }
            n202 = property on="Motor" class="Clust (strict)"("Visible"=TRUE) -> ()  [unwired: 2 in, 2 out]
            n203 = property on="Value" class="Slide (strict)"("Value"=w401, "Scale.Minimum"=w403, "Scale.Maximum"=w402, "Scale.Increment"=w400) -> ()  [unwired: 2 in, 2 out]
            n204 = property on="On/Off" class="Bool (strict)"("Visible"=w405) -> ()  [unwired: 2 in, 2 out]
            n205 = property on="Test Slider" class="Slide (strict)"("Visible"=w405) -> ()  [unwired: 2 in, 2 out]
            n206 = property on="Test Ring" class="Ring (strict)"("Visible"=w405) -> ()  [unwired: 2 in, 2 out]
            n207 = property on="Rev/Fwd" class="Clust (strict)"("Visible"=w405) -> ()  [unwired: 2 in, 2 out]
          }
          frame "Servo" {
            w417 = FALSE ("Visible")
            n208 = call <vilib>:"NT Read Number.vi"("Name"=w419) -> ("Numeric"=w418:dbl)  [unwired: 9 in, 1 out]
            n209 = property on="Test Slider" class="Slide (strict)"("Visible"=TRUE, "Scale.Maximum"=170.0 ("Scale.Range:Maximum")) -> ()  [unwired: 2 in, 2 out]
            n210 = local write "Test Slider"(w418) -> ()
            n211 = property on="Motor" class="Clust (strict)"("Visible"=w417) -> ()  [unwired: 2 in, 2 out]
            n212 = property on="Rev/Fwd" class="Clust (strict)"("Visible"=w417) -> ()  [unwired: 2 in, 2 out]
            n213 = property on="On/Off" class="Bool (strict)"("Visible"=w417) -> ()  [unwired: 2 in, 2 out]
            n214 = property on="Test Ring" class="Ring (strict)"("Visible"=w417) -> ()  [unwired: 2 in, 2 out]
          }
          frame "Relay", "Solenoid" {
            w420 = FALSE ("Visible")
            n215 = property on="Motor" class="Clust (strict)"("Visible"=w420) -> ()  [unwired: 2 in, 2 out]
            n216 = property on="Test Slider" class="Slide (strict)"("Visible"=w420) -> ()  [unwired: 2 in, 2 out]
            n217 = Search and Replace String(input string=w421, search string="/Value  **", replace string="/Direction") -> (result string=w427:string)  [unwired: 5 in, 3 out]
            n218 = property on="Test Ring" class="Ring (strict)"("Visible"=w420) -> ()  [unwired: 2 in, 2 out]
            n219 = call <vilib>:"NT Read String.vi"("Name"=w427) -> ("String"=w425:string)  [unwired: 9 in, 1 out]
            n220 = Equal?(x="Both directions", y=w425) -> (x = y?=w423:bool)
            n221 = Not(x=w423) -> (.not. x?=w424:bool)
            n222 = property on="Rev/Fwd" class="Clust (strict)"("Visible"=w423) -> ()  [unwired: 2 in, 2 out]
            n223 = property on="On/Off" class="Bool (strict)"("Visible"=w424, "Caption.Text"=w422) -> ()  [unwired: 2 in, 2 out]
          }
          frame "Compressor", "Digital Out" {
            w430 = FALSE ("Visible")
            # "Get direction and finish"
            n224 = property on="Motor" class="Clust (strict)"("Visible"=w430) -> ()  [unwired: 2 in, 2 out]
            n225 = property on="Test Slider" class="Slide (strict)"("Visible"=w430) -> ()  [unwired: 2 in, 2 out]
            n226 = property on="Test Ring" class="Ring (strict)"("Visible"=w430) -> ()  [unwired: 2 in, 2 out]
            n227 = property on="On/Off" class="Bool (strict)"("Visible"=TRUE, "Caption.Text"=w431) -> ()  [unwired: 2 in, 2 out]
            n228 = property on="Rev/Fwd" class="Clust (strict)"("Visible"=FALSE) -> ()  [unwired: 2 in, 2 out]
          }
          frame "Camera" {
            n229 = call <vilib>:"Get Last Path Segment.vi"("String in"=w438) -> ("String out"=w439:string)  [unwired: 10 in]
            n230 = property on="On/Off" class="Bool (strict)"("Visible"=FALSE) -> ()  [unwired: 2 in, 2 out]
            n231 = property on="Motor" class="Clust (strict)"("Visible"=FALSE) -> ()  [unwired: 2 in, 2 out]
            n232 = property on="Rev/Fwd" class="Clust (strict)"("Visible"=FALSE) -> ()  [unwired: 2 in, 2 out]
            n233 = case shown="\"White Balance  **\"" w439 {
              tunnel: w438 -> [w445 w454 w463 w472 w481 _ w487]
              tunnel: w437 -> [w443 w451 w460 w469 w478 _ _]
              frame "Size  **" {
                n234 = Index Array(array=w443) -> (element=w442:cluster{string[]})  [unwired: 1 in]
                n235 = call <vilib>:"NT Read String.vi"("Name"=w445) -> ("String"=w444:string)  [unwired: 9 in, 1 out]
                n236 = Unbundle(w442) -> (w440:string[])
                n237 = Match First String(2:w440, 3:w444) -> (0:w441:i32)  [unwired: 1 out]
                n238 = property on="Test Ring" class="Ring (strict)"("Value"=w441, "Strings []"=w440) -> ()  [unwired: 2 in, 2 out]
                n239 = property on="Test Ring" class="Ring (strict)"("Visible"=TRUE) -> ()  [unwired: 2 in, 2 out]
                n240 = property on="Test Slider" class="Slide (strict)"("Visible"=FALSE) -> ()  [unwired: 2 in, 2 out]
              }
              frame "White Balance  **" {
                n241 = Index Array(array=w451, index=1) -> (element=w452:cluster{string[]})
                n242 = call <vilib>:"NT Read String.vi"("Name"=w454) -> ("String"=w453:string)  [unwired: 9 in, 1 out]
                n243 = Unbundle(w452) -> (w449:string[])
                n244 = Match First String(2:w449, 3:w453) -> (0:w448:i32)  [unwired: 1 out]
                n245 = property on="Test Ring" class="Ring (strict)"("Value"=w448, "Strings []"=w449) -> ()  [unwired: 2 in, 2 out]
                n246 = property on="Test Ring" class="Ring (strict)"("Visible"=TRUE) -> ()  [unwired: 2 in, 2 out]
                n247 = property on="Test Slider" class="Slide (strict)"("Visible"=FALSE) -> ()  [unwired: 2 in, 2 out]
              }
              frame "Exposure  **" {
                n248 = Index Array(array=w460, index=2) -> (element=w461:cluster{string[]})
                n249 = call <vilib>:"NT Read String.vi"("Name"=w463) -> ("String"=w462:string)  [unwired: 9 in, 1 out]
                n250 = Unbundle(w461) -> (w457:string[])
                n251 = Match First String(2:w457, 3:w462) -> (0:w458:i32)  [unwired: 1 out]
                n252 = property on="Test Ring" class="Ring (strict)"("Value"=w458, "Strings []"=w457) -> ()  [unwired: 2 in, 2 out]
                n253 = property on="Test Ring" class="Ring (strict)"("Visible"=TRUE) -> ()  [unwired: 2 in, 2 out]
                n254 = property on="Test Slider" class="Slide (strict)"("Visible"=FALSE) -> ()  [unwired: 2 in, 2 out]
              }
              frame "Exposure Priority  **" {
                n255 = Index Array(array=w469, index=3) -> (element=w470:cluster{string[]})
                n256 = call <vilib>:"NT Read String.vi"("Name"=w472) -> ("String"=w471:string)  [unwired: 9 in, 1 out]
                n257 = Unbundle(w470) -> (w466:string[])
                n258 = Match First String(2:w466, 3:w471) -> (0:w467:i32)  [unwired: 1 out]
                n259 = property on="Test Ring" class="Ring (strict)"("Value"=w467, "Strings []"=w466) -> ()  [unwired: 2 in, 2 out]
                n260 = property on="Test Ring" class="Ring (strict)"("Visible"=TRUE) -> ()  [unwired: 2 in, 2 out]
                n261 = property on="Test Slider" class="Slide (strict)"("Visible"=FALSE) -> ()  [unwired: 2 in, 2 out]
              }
              frame "Color Enable  **" {
                n262 = Index Array(array=w478, index=4) -> (element=w479:cluster{string[]})
                n263 = call <vilib>:"NT Read String.vi"("Name"=w481) -> ("String"=w480:string)  [unwired: 9 in, 1 out]
                n264 = Unbundle(w479) -> (w475:string[])
                n265 = Match First String(2:w475, 3:w480) -> (0:w476:i32)  [unwired: 1 out]
                n266 = property on="Test Ring" class="Ring (strict)"("Value"=w476, "Strings []"=w475) -> ()  [unwired: 2 in, 2 out]
                n267 = property on="Test Ring" class="Ring (strict)"("Visible"=TRUE) -> ()  [unwired: 2 in, 2 out]
                n268 = property on="Test Slider" class="Slide (strict)"("Visible"=FALSE) -> ()  [unwired: 2 in, 2 out]
              }
              frame Default {
                n269 = property on="Test Ring" class="Ring (strict)"("Visible"=FALSE) -> ()  [unwired: 2 in, 2 out]
                n270 = property on="Test Slider" class="Slide (strict)"("Visible"=FALSE) -> ()  [unwired: 2 in, 2 out]
              }
              frame "Brightness  **", "Color Level  **", "Compression  **", "FPS  **", "Sharpness  **" {
                n271 = call <vilib>:"NT Read Number.vi"("Name"=w487) -> ("Numeric"=w486:dbl)  [unwired: 9 in, 1 out]
                n272 = local write "Test Slider"(w486) -> ()
                n273 = property on="Test Slider" class="Slide (strict)"("Visible"=TRUE, "Scale.Maximum"=100.0 ("Scale.Range:Maximum")) -> ()  [unwired: 2 in, 2 out]
                n274 = property on="Test Ring" class="Ring (strict)"("Visible"=FALSE) -> ()  [unwired: 2 in, 2 out]
              }
            }
          }
        }
        n275 = property on="Progress" class="Clust (strict)"("Visible"=FALSE) -> ()  [unwired: 2 in, 2 out]
      }
      event "Test Name": Mouse Enter {
        # "Populate the ring with the list of tests"
        n276 = event-data() -> ()  [unwired: 1 in, 1 out]
        n277 = call <vilib>:"NT Read String Array.vi"("Name"="TestMode/TestList") -> ("String Array"=w495:string[])  [unwired: 9 in, 1 out]
        n278 = Build Array (concatenate)("Select the test to run...", w495) -> (w494:string[])
        n279 = property on="Test Name" class="Ring (strict)"("Strings []"=w494) -> ()  [unwired: 2 in, 2 out]
      }
      event "Test Name": Value Change {
        w497 = FALSE ("Visible")
        # "Tell the robot the test name to run"
        n280 = event-data() -> ("NewVal"=w501:u16)  [unwired: 1 in]
        n281 = property on="Test Name" class="Ring (strict)"() -> ("Strings []"=w502:string[])  [unwired: 2 in, 2 out]
        n282 = local write "Progress"(T15 {"Test Progress"=0, "Test Progress Text"=""} ("Progress")) -> ()
        n283 = Index Array(array=w502, index=w501) -> (element=w500:string)
        n284 = call <vilib>:"NT Write String.vi"("String"=w500, "Name"="TestMode/TestName") -> ()  [unwired: 9 in, 1 out]
        n285 = property on="Progress" class="Clust (strict)"("Visible"=TRUE) -> ()  [unwired: 2 in, 2 out]
        n286 = property on="Motor" class="Clust (strict)"("Visible"=w497) -> ()  [unwired: 2 in, 2 out]
        n287 = property on="Test Slider" class="Slide (strict)"("Visible"=w497) -> ()  [unwired: 2 in, 2 out]
        n288 = property on="On/Off" class="Bool (strict)"("Visible"=w497) -> ()  [unwired: 2 in, 2 out]
        n289 = property on="Rev/Fwd" class="Clust (strict)"("Visible"=w497) -> ()  [unwired: 2 in, 2 out]
        n290 = property on="Test Ring" class="Ring (strict)"("Visible"=w497) -> ()  [unwired: 2 in, 2 out]
      }
      event "Listbox": Double Click {
        n291 = event-data() -> ("PlatMods.Shift"=w505:bool, "Row"=w507:i32)  [unwired: 1 in]
        n292 = case shown="True" w505 {
          tunnel: w507 -> [w511 _]
          tunnel: 1 -> [w510 _]
          frame False {
            n293 = property on="Listbox" class="LstBox (strict)"() -> ("Item Symbols"=w509:i32[])  [unwired: 2 in, 2 out]
            n294 = Replace Array Subset(array=w509, new element=w510, index=w511) -> (w508:i32[])
            n295 = property on="Listbox" class="LstBox (strict)"("Item Symbols"=w508) -> ()  [unwired: 2 in, 2 out]
          }
          frame True {
            w512 = 0 ("Top Row")
            n296 = property on="Listbox" class="LstBox (strict)"() -> ("Number of Rows"=w514:u32)  [unwired: 2 in, 2 out]
            n297 = Initialize Array(0, w514) -> (w513:i32[])
            n298 = property on="Listbox" class="LstBox (strict)"("Top Row"=w512, "Value"=w512, "Item Symbols"=w513) -> ()  [unwired: 2 in, 2 out]
          }
        }
      }
      event "Listbox": Key Down {
        n299 = event-data() -> ("VKey"=w518:T28)  [unwired: 1 in]
        n300 = case shown="\"Left\", \"Right\"" w518 {
          selector: w518 -> [w523 _]
          tunnel: eventvkey."Left" ("VKey") -> [w521 _]
          frame "Left", "Right" {
            n301 = Equal?(x=w521, y=w523) -> (x = y?=w522:bool)
            n302 = Select(t=0, s=w522, f=1) -> (s? t:f=w524:i32)
            n303 = property on="Listbox" class="LstBox (strict)"() -> ("Item Symbols"=w527:i32[])  [unwired: 2 in, 2 out]
            n304 = Replace Array Subset(array=w527, new element=w524, index="Listbox") -> (w526:i32[])
            n305 = property on="Listbox" class="LstBox (strict)"("Item Symbols"=w526) -> ()  [unwired: 2 in, 2 out]
          }
          frame Default {
          }
        }
      }
      event "DB Camera Config": Value Change {
        n306 = event-data() -> ("NewVal"=w531:bool)  [unwired: 1 in]
        n307 = case shown="False" w531 {
          tunnel: w530 -> [w540 _]
          tunnel: [w533 w551] -> w529
          tunnel: w528 -> [w532 w551]
          frame False {
            w547 = "Camera"
            w550 = FALSE ("Visible")
            n308 = local read "Camera Settings"() -> (w539:T7)
            n309 = Index Array(array=w540) -> (element=w543:cluster{string[]})  [unwired: 1 in]
            n310 = Unbundle(w539) -> ("Frame Rate"=w538:i32, "Compression"=w537:i32, "Size"=w541:u16)
            n311 = Unbundle(w543) -> (w542:string[])
            n312 = Index Array(array=w542, index=w541) -> (element=w536:string)
            n313 = call-poly <vilib>:"Write Key.vi"("section"=w547, "value"=w536, "key"="Size", "refnum"=w532) -> ("refnum out"=w549:T21)  [unwired: 2 in, 5 out]
            n314 = call-poly <vilib>:"Write Key.vi"("section"=w547, "value"=w538, "key"="FrameRate", "refnum"=w549) -> ("refnum out"=w548:T21)  [unwired: 1 in, 6 out]
            n315 = property on="Camera Settings" class="Clust (strict)"("Visible"=w550) -> ()  [unwired: 2 in, 2 out]
            n316 = local write "DB Camera Config"(w550) -> ()
            n317 = call-poly <vilib>:"Write Key.vi"("section"=w547, "value"=w537, "key"="Compression", "refnum"=w548) -> ("refnum out"=w534:T21)  [unwired: 1 in, 6 out]
            n318 = call <vilib>:"Close Config Data.vi"("refnum"=w534) -> ("file path"=w535:path)  [unwired: 2 in, 8 out]
            n319 = call <vilib>:"Open Config Data.vi"("configuration file path"=w535) -> ("refnum"=w533:T21)  [unwired: 8 in, 2 out]
          }
          frame True {
            n320 = property on="Camera Settings" class="Clust (strict)"("Visible"=TRUE) -> ()  [unwired: 2 in, 2 out]
          }
        }
      }
      event "Camera Settings": Value Change {
        n321 = event-data() -> ("NewVal"=w564:T7)  [unwired: 1 in]
        n322 = Index Array(array=w560) -> (element=w559:cluster{string[]})  [unwired: 1 in]
        n323 = Unbundle(w564) -> ("Frame Rate"=w555:i32, "Compression"=w554:i32, "Size"=w557:u16)
        n324 = Unbundle(w559) -> (w558:string[])
        n325 = Index Array(array=w558, index=w557) -> (element=w556:string)
        n326 = Format Into String(format string="%s   %dfps   %d%%", w556, w555, w554) -> (resulting string=w561:string)  [unwired: 2 in, 1 out]
        n327 = Build Array(w561) -> (w562:string[])
        n328 = property on="DB Camera Config" class="Bool (strict)"("Strings [4]"=w562) -> ()  [unwired: 2 in, 2 out]
      }
      event "Motor.Enable": Value Change {
        n329 = event-data() -> ("NewVal"=w570:bool)  [unwired: 1 in]
        n330 = Unbundle("Motor") -> ("Value"=w569:dbl)  [unwired: 1 out]
        n331 = Select(t=w569, s=w570, f=0.0) -> (s? t:f=w567:dbl)
        n332 = call <vilib>:"NT Write Number.vi"("Numeric"=w567, "Name"=w566) -> ()  [unwired: 9 in, 1 out]
      }
      event "Test Slider": Value Change {
        n333 = event-data() -> ("NewVal"=w573:dbl)  [unwired: 1 in]
        n334 = call <vilib>:"NT Write Number.vi"("Numeric"=w573, "Name"=w574) -> ()  [unwired: 9 in, 1 out]
      }
      event "On/Off": Value Change {
        n335 = event-data() -> ("NewVal"=w578:bool)  [unwired: 1 in]
        n336 = Boolean To (0,1)(Boolean=w578) -> (0, 1=w577:i16)
        n337 = call <vilib>:"NT Write Number.vi"("Numeric"=w577, "Name"=w576) -> ()  [unwired: 9 in, 1 out]
      }
      event "Rev/Fwd": Value Change {
        n338 = event-data() -> ("NewVal.Forward"=w586:bool, "NewVal.Reverse"=w585:bool)  [unwired: 1 in]
        n339 = Boolean To (0,1)(Boolean=w586) -> (0, 1=w582:i16)
        n340 = Boolean To (0,1)(Boolean=w585) -> (0, 1=w584:i16)
        n341 = Negate(x=w584) -> (-x=w583:i16)
        n342 = Add(x=w582, y=w583) -> (x+y=w581:i16)
        n343 = call <vilib>:"NT Write Number.vi"("Numeric"=w581, "Name"=w580) -> ()  [unwired: 9 in, 1 out]
      }
      event "Test Ring": Value Change {
        n344 = event-data() -> ("NewVal"=w590:u16)  [unwired: 1 in]
        n345 = property on="Test Ring" class="Ring (strict)"() -> ("Strings []"=w591:string[])  [unwired: 2 in, 2 out]
        n346 = Index Array(array=w591, index=w590) -> (element=w589:string)
        n347 = call <vilib>:"NT Write String.vi"("String"=w589, "Name"=w588) -> ()  [unwired: 9 in, 1 out]
      }
      event "Rec Mode": Value Change {
        # "Update globals for recording mode and path to read log from.\nClear when logging and let NetworkTables set path for vision to\nuse."
        n348 = event-data() -> ("NewVal"=w601:enum32{"Stop", "Record", "Playback"})  [unwired: 1 in]
        n349 = global write "WPI_DashboardLogging Global.vi" "Logging Filename"(path "") -> ()
        n350 = case shown="\"Stop\", \"Record\"" w601 {
          tunnel: w600 -> [_ w603 w611]
          tunnel: [_ _ w610] -> w597
          tunnel: [_ _ w609] -> _
          tunnel: w595 -> [_ _ w607]
          tunnel: cluster{i32, i32} {-250, 170} -> [_ _ w606]
          tunnel: [_ _ T29 {"Image Size"=TRUE, "Image Type"=TRUE, "Pixel Value"=TRUE, "ROI Information"=TRUE, "Zoom Factor"=FALSE} ("Image Information Shown:All Elements")] -> w593
          tunnel: [_ _ TRUE ("Zoom Factor")] -> w592
          frame Default {
          }
          frame "Stop", "Record" {
            # "Place Window too"
            n351 = invoke class="VI" method="FP.Close"(reference=w603) -> (reference out=w602:refnum<vi>)  [unwired: 2 in, 2 out]
            n352 = invoke class="VI" method="Abort VI"(reference=w602) -> ()  [unwired: 2 in, 3 out]
          }
          frame "Playback" {
            n353 = call "Open Playback Panel.vi"("Offset"=w606, "DB VI Ref"=w607, "Playback in"=w611) -> ("Playback out"=w608:refnum<vi>)  [unwired: 8 in]
            n354 = register-events(w608) -> (reference out=w610:refnum<event-registration>, error out=w609:errorcluster)  [unwired: 2 in]
          }
        }
        n355 = global write "WPI_DashboardLogging Global.vi" "Recording"(w601) -> ()
        n356 = property on="Camera Image" class="ImageControl"("Image Information Shown"=w593, "Image Information Visible"=w592) -> ()  [unwired: 2 in, 2 out]
        n357 = call <vilib>:"WPI_DashboardNT Log FieldName Cache.vi"("Operation"=enum16{"Lookup/Add", "Index", "Clear"}."Clear") -> ()  [unwired: 8 in, 3 out]
      }
      event Panel Close {
        w612 = enum32{"Stop", "Record", "Playback"}."Stop" ("Rec Mode")
        n358 = event-data() -> ()  [unwired: 1 in, 4 out]
        n359 = local write "Rec Mode"(w612) -> ()
        n360 = global write "WPI_DashboardLogging Global.vi" "Recording"(w612) -> ()
      }
      event Panel Close {
        # "Abort playback window and ourself"
        n361 = event-data() -> ()  [unwired: 1 in, 4 out]
        n362 = invoke class="VI" method="FP.Close"(reference=w617) -> (reference out=w616:refnum<vi>)  [unwired: 2 in, 2 out]
        n363 = invoke class="VI" method="Abort VI"(reference=w616) -> (error out=w615:errorcluster)  [unwired: 2 in, 2 out]
        n364 = invoke class="VI" method="Abort VI"(error in=w615) -> ()  [unwired: 2 in, 3 out]
      }
    }
  }
  n365 = property on="On/Off" class="Bool (strict)"("Visible"=w29) -> ()  [unwired: 2 in, 2 out]
  n366 = property on="Motor" class="Clust (strict)"("Visible"=w29) -> ()  [unwired: 2 in, 2 out]
  n367 = property on="Progress" class="Clust (strict)"("Visible"=w29) -> ()  [unwired: 2 in, 2 out]
  n368 = property on="Test Ring" class="Ring (strict)"("Visible"=w29) -> ()  [unwired: 2 in, 2 out]
  n369 = property on="Rev/Fwd" class="Clust (strict)"("Visible"=w29) -> ()  [unwired: 2 in, 2 out]
  n370 = property on="Camera Settings" class="Clust (strict)"("Visible"=w29) -> ()  [unwired: 2 in, 2 out]
  n371 = local write "DB Camera Config"(w29) -> ()
  n372 = global write "WPI_DashboardLogging Global.vi" "Recording"(w12) -> ()
  n373 = local write "Rec Mode"(w12) -> ()
